vi "Load Linked List.vi"(6 "Persistence":refnum<class "IPersist.lvclass">, 7 "Parent ID":string, 8 "error in (no error)":errorcluster, 10 "File Path":path, 11 "Linked List":refnum<class "ILinked List.lvclass">) -> (0 "error out":errorcluster, 3 "Linked List Ref out":refnum<data-value>, 5 "Linked List ID out":string)   [LabVIEW 2020, in "Linked Lists.lvlib" / "Linked List Ref.lvclass"]
uses:
  <vilib>/gpm_packages/@cs/linked-list/Source/Linked List/Linked List Ref/Linked List Ref.lvclass
  <vilib>/gpm_packages/@cs/linked-list/Source/Linked List/ILinkedList/ILinked List.lvclass
  <vilib>/gpm_packages/@cs/persistence/source/IPersist/IPersist.lvclass
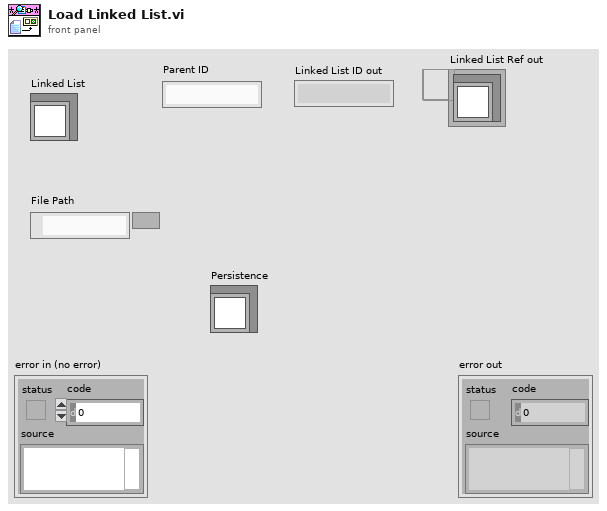
[diagram p1: front panel]
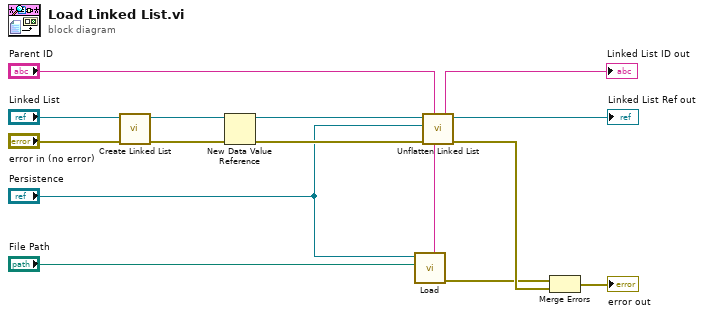
[diagram p0: block diagram]
diagram:
  n1 = call-dynamic "Create Linked List.vi"("error in (no error)"="error in (no error)", "ILinked List in"="Linked List") -> ("error out"=w8:errorcluster, "ILinked List out"=w5:refnum<class "ILinked List.lvclass">)  [unwired: 8 in]
  n2 = New Data Value Reference(data value=w5, error in=w8) -> (data value reference=w10:refnum<data-value>, error out=w9:errorcluster)
  n3 = call-dynamic "Load.vi"("Path"="File Path", "IPersist in"="Persistence") -> ("error out"=w1:errorcluster, "Flattened String"=w2:string)  [unwired: 7 in, 1 out]
  n4 = call <vilib>:"Unflatten Linked List.vi"("Flattened Linked List"=w2, "Parent ID"="Parent ID", "error in (no error)"=w9, "Persistence"="Persistence", "Linked List Ref"=w10) -> ("error out"=w13:errorcluster, "Linked List Ref out"=→"Linked List Ref out":refnum<data-value>, "Linked List ID out"=→"Linked List ID out":string)  [unwired: 4 in]
  n5 = Merge Errors(w1, w13) -> (→"error out":errorcluster)
